vi "Write Status 1D.vi"(8 "error in (no error)":errorcluster, 10 "statuses":T1[](array[typedef]) {"duration" format="%d us"}, 11 "status pointer in":refnum<class "Status.lvclass">) -> (0 "error out":errorcluster, 3 "status pointer out":refnum<class "Status.lvclass">)   [LabVIEW 2017, in "DSF Core.lvlib" / "Status.lvclass"]
uses:
  Status.lvclass
  C:/Git/DSF/LabVIEW-Memory/Source/Classes/Pointer/Pointer.lvclass
  Status/Status Data.ctl
  LabVIEW-Memory/Source/Classes/Pointer/Pointer.lvclass
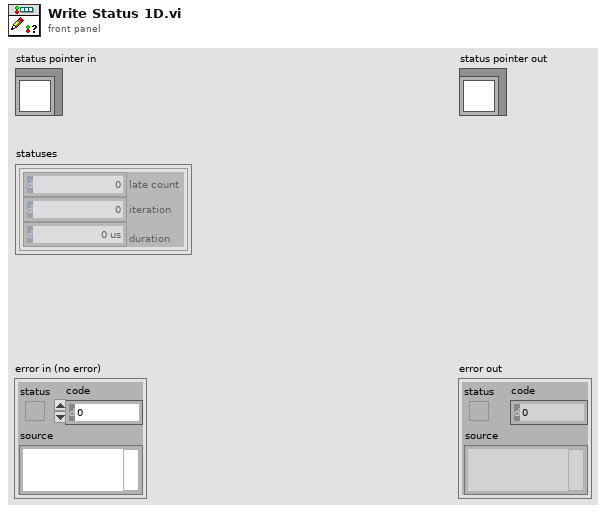
[diagram p1: front panel]
types:
  T1 = typedef "DSF Core.lvlib/Status.lvclass/Status Data.ctl" = cluster{"late count":u64, "iteration":u64, "duration":u32}
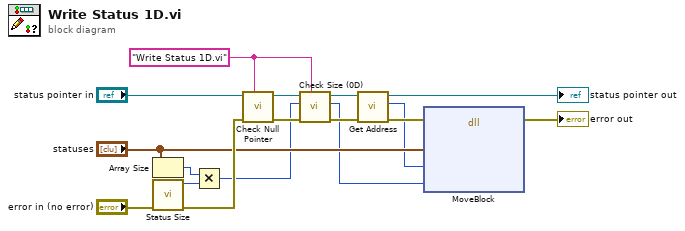
[diagram p0: block diagram]
diagram:
  w11 = "Write Status 1D.vi" ("source vi name")
  n1 = Array Size(array="statuses") -> (size(s)=w6:i32)
  n2 = call "Status Size.vi"("error in (no error)"="error in (no error)") -> ("error out"=w8:errorcluster, "size"=w7:u64)  [unwired: 9 in]
  n3 = Multiply(x=w6, y=w7) -> (x*y=w3:u64)
  n4 = call "Check Null Pointer.vi"("source vi name"=w11, "error in (no error)"=w8, "Pointer in"="status pointer in") -> ("error out"=w9:errorcluster, "Pointer out"=w14:refnum<class "Status.lvclass">)  [unwired: 7 in]
  n5 = call "Check Size (0D).vi"("source vi name"=w11, "error in (no error)"=w9, "required size"=w3, "Pointer in"=w14) -> ("error out"=w5:errorcluster, "required size out"=w2:u64, "Pointer out"=w12:refnum<class "Status.lvclass">)  [unwired: 5 in]
  n6 = call "Get Address.vi"("Pointer in"=w12) -> ("address"=w1:u64, "Pointer out"=→"status pointer out":refnum<class "Status.lvclass">)  [unwired: 9 in]
  n7 = dll-call lib="LabVIEW" fn="MoveBlock"(error in=w5, "src"="statuses", "dst"=w1, "size"=w2) -> (error out=→"error out":errorcluster)  [unwired: 6 in, 1 out]
